vi "Vision Research Phantom Series PhInt PhImHisto.vi"(0 "pBMIH":T2, 1 "pPixel In":u16[](array[numeric]), 2 "HistoSize":u32, 3 "Color":T1, 5 "Error In (no error)":errorcluster) -> (14 "pHisto":u32[](array[numeric]), 15 "pAvgR":u32, 16 "pAvgG":u32, 17 "pAvgB":u32, 19 "Error Out":errorcluster)   [LabVIEW 2013, in "VRI.lvlib"]
doc: "PhInt.dll\n\nPhImHisto\nvoid PhImHisto(PBITMAPINFOHEADER pBMIH, PBYTE pPixel, UINT HistoSize, UINT Color, PUINT pHisto, \n PUINT PAvgR, PUINT pAvgG, PUINT pAvgB);\n\nParameters Description\npBMIH Header of the image.\npPixel Pixel Array of the image.\nHistoSize Dimension of the histogram array. Can be less than the number of the possible levels of \n the selected color; in this case, a number of counts for neighbor levels are accumulated in \n the same histogram value.\nColor Compute the histogram on this selected color: 0 = rgb converted to gray, 1 = red, \n 2 = green, 3 = blue\npHisto The result: an array of integers that count the occurance of each level or set of levels \n (if HistoSize < maximum value of the pixel)\npAvgR, Optional results (not cumputed if pointers are NULL). The average of the RGB \npAvgG, color components on the full image.\npAvgR \nReturn void\nComments PhImHisto computes the histogram of an image"
uses:
  VRI.lvlib
  _Type Defs/BITMAPINFOHEADER.ctl
  _Type Defs/PhInt Color.ctl
  Phantom DLLs/PhInt.dll
panel:
  # "For instructions on the use of this VI, press Ctrl+H to display the help window and move the mouse over the icon, controls, and indicators"
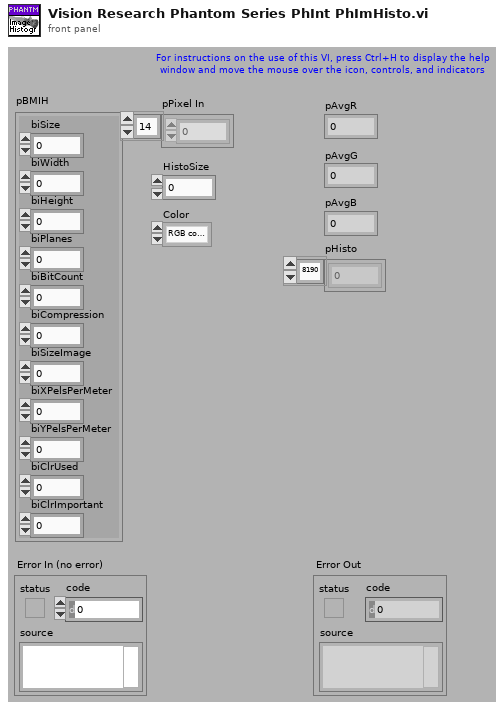
[diagram p1: front panel]
types:
  T1 = typedef "VRI.lvlib/PhInt Color.ctl" = enum32{"RGB converted to gray", "RED", "GREEN", "BLUE"}
  T2 = typedef "VRI.lvlib/BITMAPINFOHEADER.ctl" = cluster{"biSize":u32, "biWidth":i32, "biHeight":i32, "biPlanes":u16, "biBitCount":u16, "biCompression":u32, "biSizeImage":u32, "biXPelsPerMeter":i32, "biYPelsPerMeter":i32, "biClrUsed":u32, "biClrImportant":u32}
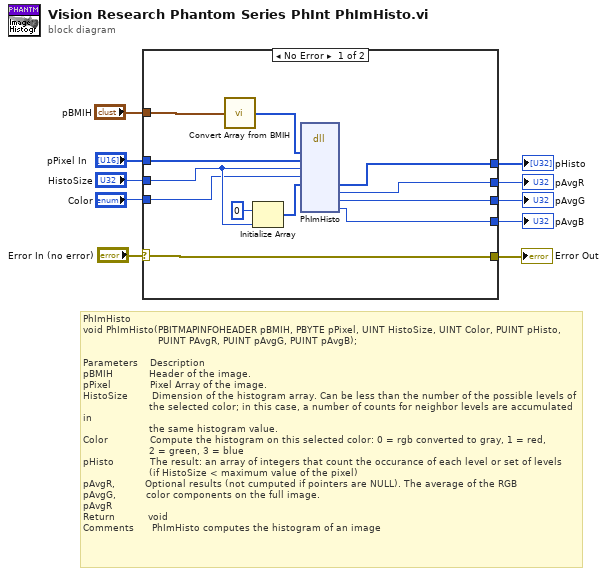
[diagram p0: block diagram]
diagram:
  # "PhImHisto\nvoid PhImHisto(PBITMAPINFOHEADER pBMIH, PBYTE pPixel, UINT HistoSize, UINT Color, PUINT pHisto, \n                         PUINT PAvgR, PUINT pAvgG, PUINT pAvgB);\n\nParameters    Description\npBMIH            Header of the image.\npPixel             Pixel Array of the image.\nHistoSize        Dimension of the histogram array. Can be less than the number of the possible levels of  \n                      the selected color; in this case, a number of counts for neighbor levels are accumulated in \n                      the same histogram value.\nColor              Compute the histogram on this selected color: 0 = rgb converted to gray, 1 = red, \n                      2 = green, 3 = blue\npHisto            The result: an array of integers that count the occurance of each level or set of levels \n                      (if HistoSize < maximum value of the pixel)\npAvgR,          Optional results (not cumputed if pointers are NULL). The average of the RGB \npAvgG,          color components on the full image.\npAvgR                                      \nReturn           void\nComments      PhImHisto computes the histogram of an image"
  n1 = case shown="No Error" "Error In (no error)" {
    selector: "Error In (no error)" -> [w22 w23]
    tunnel: [w22 w23] -> w9
    tunnel: "pBMIH" -> [w21 _]
    tunnel: "pPixel In" -> [w20 _]
    tunnel: [w19 _] -> w6
    tunnel: [w18 _] -> w5
    tunnel: [w17 _] -> w4
    tunnel: "HistoSize" -> [w16 _]
    tunnel: "Color" -> [w15 _]
    tunnel: [w14 _] -> w2
    frame No Error {
      n2 = call "Convert Array from BMIH.vi"("BITMAPINFOHEADER"=w21) -> ("Array"=w13:u8[])
      n3 = Initialize Array(u32 0 ("element"), w16) -> (w11:u32[])
      n4 = dll-call lib="C:/Projects/SDK/32-bit/Vision Research Phantom Series Labview Driver/Phantom DLLs/PhInt.dll" fn="PhImHisto"("pBMIH"=w13, "pPixel"=w20, "HistoSize"=w16, "Color"=w15, "pHisto"=w11) -> ("pHisto"=w14:u32[], "pAvgR"=w19:u32, "pAvgG"=w18:u32, "pAvgB"=w17:u32)  [unwired: 6 in, 7 out]
    }
    frame Error {
    }
  }
  "Error Out" <- w9
  "pAvgR" <- w6
  "pAvgG" <- w5
  "pAvgB" <- w4
  "pHisto" <- w2
